vi "Double to Integer.vi"(1 "DBL Array":cdb[](array[numeric])) -> (0 "I32 Array":cdb[](array[numeric]))   [LabVIEW 2018]
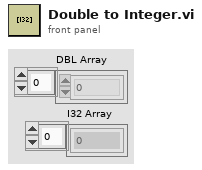
[diagram p1: front panel]
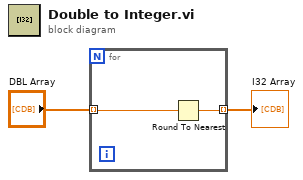
[diagram p0: block diagram]
diagram:
  n1 = for {
    tunnel: "DBL Array" -> [w3] mode=indexing
    tunnel: [w4] -> w1 mode=indexing
    n2 = Round To Nearest(number=w3) -> (nearest integer value=w4:cdb)
  }
  "I32 Array" <- w1
